vi "SynchRefs.vi"() -> ()   [LabVIEW 2020]
uses:
  NAI5330A_TypeDefs.llb/NAI5330A_Command.ctl
  NAI5330A_TypeDefs.llb/NAI5330A_VI_Window_Position.ctl
panel:
  in  "ActiveChannel":refnum<notifier>
  in  "VI.Window.Pos":refnum<notifier>
  in  "Tab.Main.SelectedPage":refnum<notifier>
  in  "Tab.Main.PrevPage":refnum<notifier>
  in  "Tab.Main.Ref":refnum<notifier>
  in  "Instr.Settings.Ref":refnum<notifier>
  in  "Command.Value.2":refnum<notifier>
  in  "Ch2.AveAngleReadings":refnum<notifier>
  in  "Ch1.AveAngleReadings":refnum<notifier>
  in  "UpdateTime.Ref.Parameters":refnum<notifier>
  in  "UpdateTime.Degrees":refnum<notifier>
  in  "Angle.Difference":refnum<notifier>
  in  "Command.Execution.Status":refnum<notifier>
  in  "Command.MonitorInstr.Responce":refnum<notifier>
  in  "Command.Value1":refnum<notifier>
  in  "Command":refnum<queue>
  in  "SynchRefs":T1
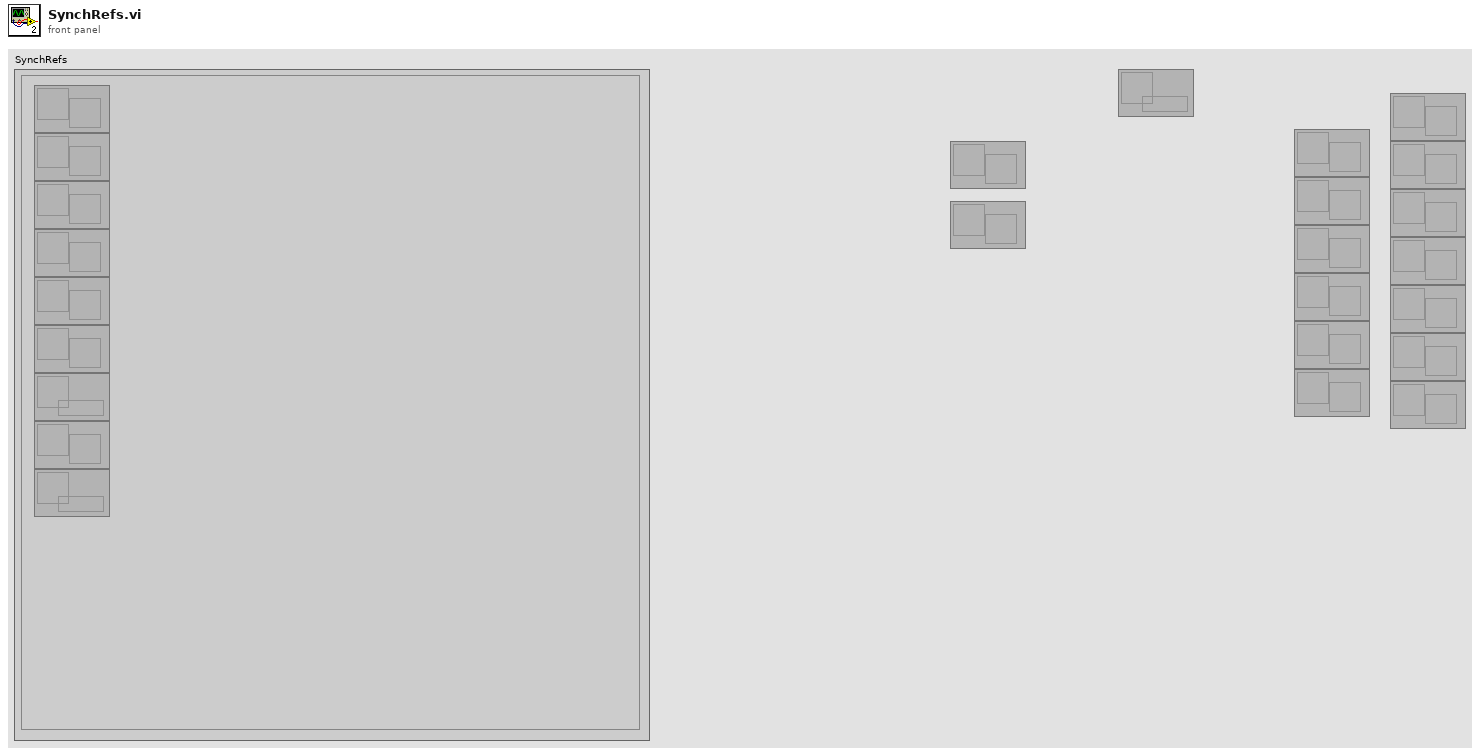
[diagram p1: front panel]
types:
  T1 = cluster{"EXIT":refnum<notifier>, "UDP.IP.Address":refnum<notifier>, "UDP.LocalPort.Write":refnum<notifier>, "UDP.Port.Read":refnum<notifier>, "UDP.ExecEng.Command":refnum<notifier>, "UDP.ExecEng.Port.Receiver":refnum<notifier>, "UDP.Instrument.Instruction":refnum<queue>, "UDP.ExecEng.Command.String.Monitor":refnum<notifier>, "UDP.Instrument.Responce.Q":refnum<queue>}
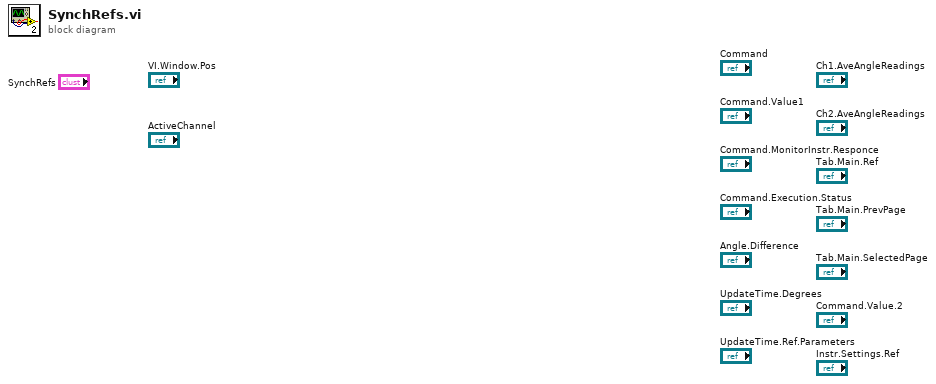
[diagram p0: block diagram]
diagram:
